vi "Letters_input.vi"() -> (1 "output cluster":T6)   [LabVIEW 2009]
panel:
  out "TRJs":T1
  in  "Element In":T2
  out "Elements Out":T3(array[cluster])
  out "Init Cluster":T4
  in  "Type":i32
  out "error out":errorcluster
  in  "error in (no error)":errorcluster
  in  "Outputmode":u16(ring) items=["Get Path", "Make Layout", "Create TRJs"]
  in  "Tab Control":enum32{"Main", "Expert", "Output"}(tab)
  in  "String of machining charactors":string
  in  "change size factor\nheight=1mm*factor\nwidth=0.5mm*factor":dbl=1.0
  in  "interval of charactors (X)\n\"-\" right; \"+\" left":dbl=-0.7
  in  "interval of charactors (Y)\n\"-\"down; \"+\" up":dbl
  in  "Initial position":dbl[](array[numeric])=[24.39, -7.31] format="%.6f"
  in  "stop":bool
  in  "XY Line Arc trj":T5={"Velocity (units/s)"=3.0, "Acceleration (unts/s2)"=50.0, "Number of times of execution"=1} {"Acceleration (unts/s2)" format="%.6f"; "Velocity (units/s)" format="%.6f"; "Number of times of execution" format="%.6f"}
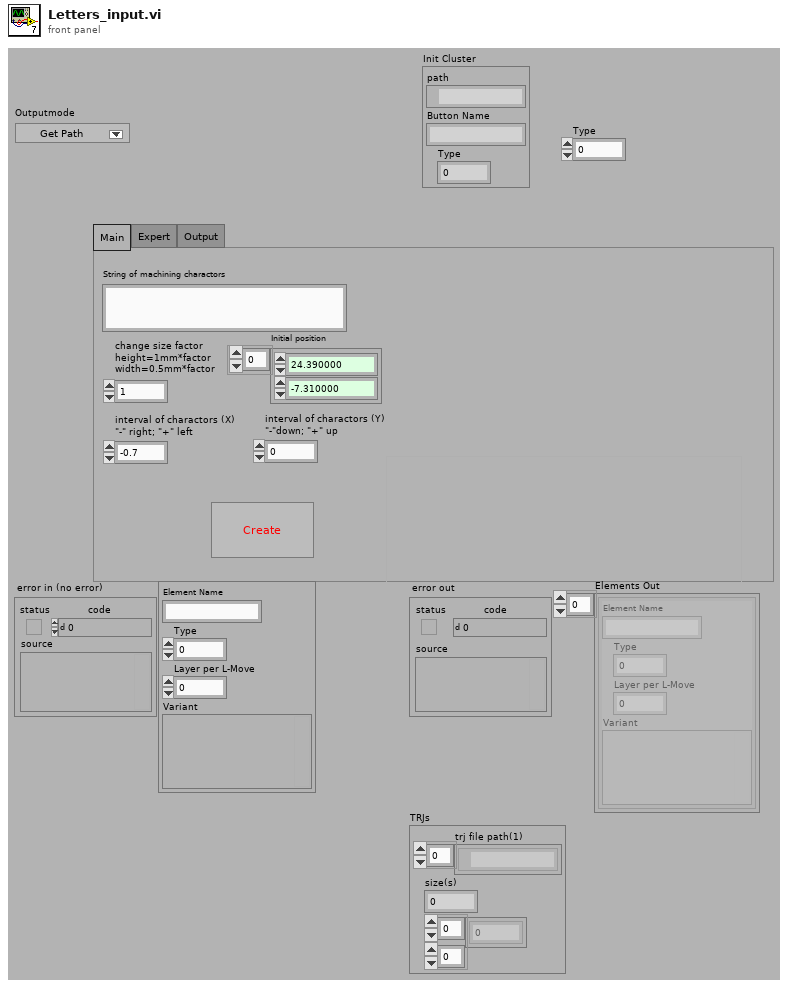
[diagram p1: front panel]
types:
  T1 = cluster{"trj file path(1)":path[], "size(s)":i32, dbl[][]}
  T2 = cluster{"Element Name":string, "Type":i32, "Layer per L-Move":i32, "Variant":variant}
  T3 = cluster{"Element Name":string, "Type":i32, "Layer per L-Move":i32, "Variant":variant}[]
  T4 = cluster{"path":path, "Button Name":string, "Type":i32}
  T5 = cluster{"Velocity (units/s)":dbl, "Acceleration (unts/s2)":dbl, "Number of times of execution":i32}
  T6 = cluster{"Initial position":dbl[], "interval of charactors (Y)\n\"-\"down; \"+\" up":dbl, "interval of charactors (X)\n\"-\" right; \"+\" left":dbl, "change size factor\nheight=1mm*factor\nwidth=0.5mm*factor":dbl, "String of machining charactors":string, "XY Line Arc trj":cluster{"Velocity (units/s)":dbl, "Acceleration (unts/s2)":dbl, "Number of times of execution":i32}}
  T7 = cluster{"Element Name":string, "Value":i32, "Layer per L-Move":i32, "Variant":variant}
  T8 = cluster{"Element Name":string, "Value":i32, "Layer per L-Move":i32, "Variant":variant}[]
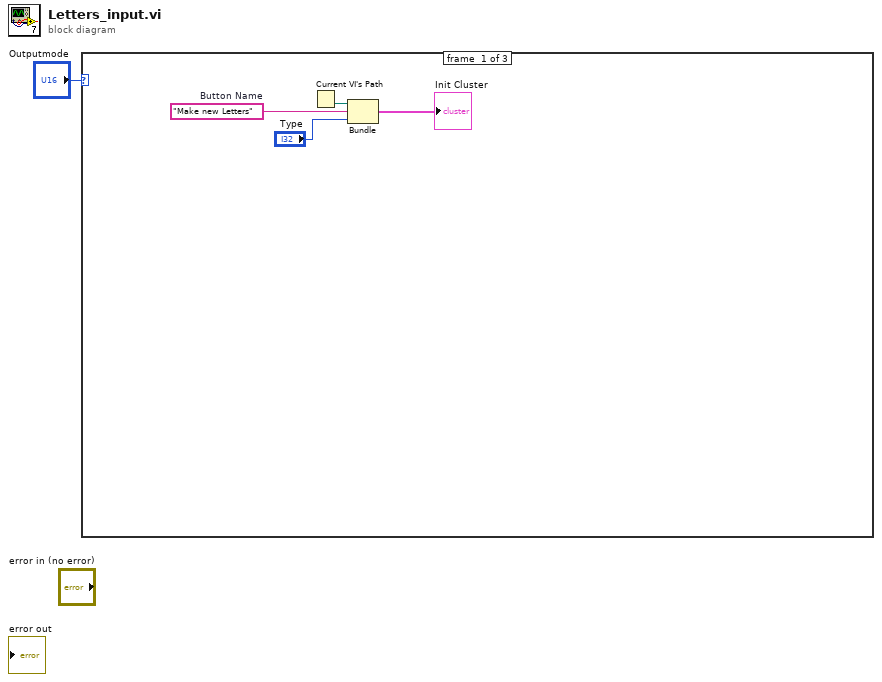
[diagram p0: block diagram]
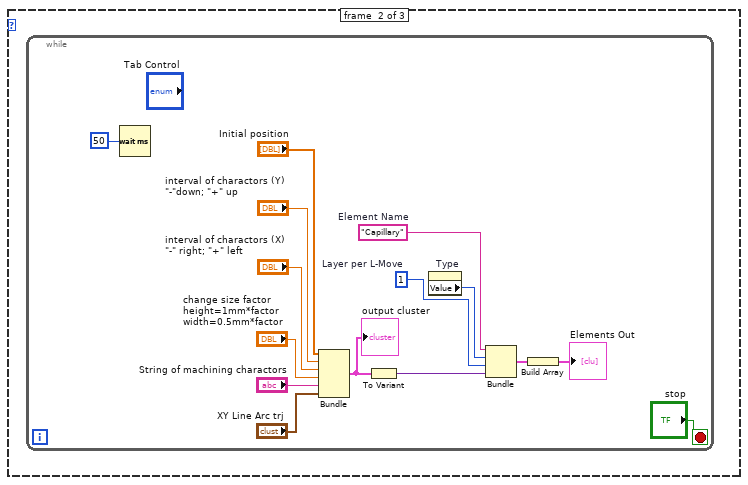
[diagram p2: hidden frame]
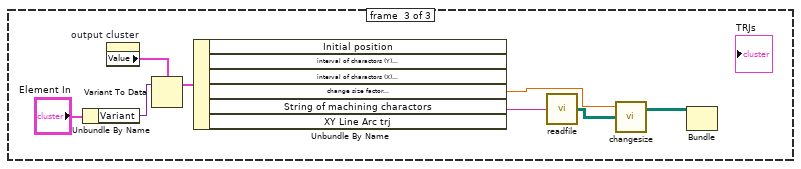
[diagram p3: hidden frame]
diagram:
  n1 = case shown="2" "Outputmode" {
    frame #0 {
      w3 = "Make new Letters"  # Button Name
      n2 = Current VI's Path() -> (path=w2:path)
      n3 = Bundle("path"=w2, "Button Name"=w3, "Type"="Type") -> (→"Init Cluster":T4)  [unwired: 1 in]
    }
    frame #1 {
      n4 = while {
        stop <- "stop" stop-if-true
        w9 = 1  # Layer per L-Move
        w10 = "Capillary"  # Element Name
        n5 = Wait (ms)(milliseconds to wait=u32 50) -> ()  [unwired: 1 out]
        n6 = Bundle("Initial position"="Initial position", "interval of charactors (Y)\n\"-\"down; \"+\" up"="interval of charactors (Y)\n\"-\"down; \"+\" up", "interval of charactors (X)\n\"-\" right; \"+\" left"="interval of charactors (X)\n\"-\" right; \"+\" left", "change size factor\nheight=1mm*factor\nwidth=0.5mm*factor"="change size factor\nheight=1mm*factor\nwidth=0.5mm*factor", "String of machining charactors"="String of machining charactors", "XY Line Arc trj"="XY Line Arc trj") -> (w12:T6)  [unwired: 1 in]
        "output cluster" <- w12
        n7 = To Variant(anything=w12) -> (Variant=w11:variant)
        n8 = property on="Type" class="DigNum (strict)"() -> ("Value"=w8:i32)  [unwired: 2 in, 2 out]
        n9 = Bundle("Element Name"=w10, "Value"=w8, "Layer per L-Move"=w9, "Variant"=w11) -> (w7:T7)  [unwired: 1 in]
        n10 = Build Array(w7) -> (→"Elements Out":T8)
      }
    }
    frame #2 {
      n11 = Unbundle By Name("Element In") -> ("Variant"=w26:variant)
      n12 = property on="output cluster" class="Clust (strict)"() -> ("Value"=w27:T6)  [unwired: 2 in, 2 out]
      n13 = Variant To Data(Variant=w26, type=w27) -> (data=w25:T6)  [unwired: 1 in, 1 out]
      n14 = Unbundle By Name(w25) -> ("change size factor\nheight=1mm*factor\nwidth=0.5mm*factor"=w23:dbl, "String of machining charactors"=w24:string)  [unwired: 4 out]
      n15 = call "readfile.vi"("String"=w24) -> ("array for path"=w22:path[][])  [unwired: 4 out]
      n16 = call "changesize.vi"("array for path"=w22, "x"=w23) -> ("changed size file path array"=w21:path[][])  [unwired: 2 out]
      n17 = Bundle("changed size file path array"=w21) -> ()  [unwired: 3 in, 1 out]
    }
  }
